vi "Get Meta Data.vi"   [LabVIEW 2015, in "NI STM.lvlib"]
doc: "Returns the meta data associated with the STM session.\n\nCopyright 2015, 2016, 2017 National Instruments Corporation\n\nLicensed under the Apache License, Version 2.0 (the \"License\"); you may not use this file except in compliance with the License.\n\n You may obtain a copy of the License at\n\n http://www.apache.org/licenses/LICENSE-2.0\n\nUnless required by applicable law or agreed to in writing, software distributed under the License is distributed on an \"AS IS\" BASIS, WITHOUT WARRANTIES OR CONDITIONS OF ANY KIND, either express or implied.\n\nSee the License for the specific language governing permissions and limitations under the License."
uses:
  <vilib>/NI/STM/NI STM.lvlib
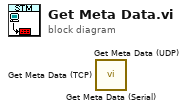
[diagram p0: block diagram]
diagram:
  n1 = call <vilib>:"Get Meta Data (Serial).vi"() -> ()  [unwired: 9 in, 3 out]
  n2 = call <vilib>:"Get Meta Data (UDP).vi"() -> ()  [unwired: 9 in, 3 out]
  n3 = call <vilib>:"Get Meta Data (TCP).vi"() -> ()  [unwired: 9 in, 3 out]
